vi "Convert to Range.vi"(1 "Output Level (1.0 mA)":dbl) -> (0 "Current Range (0: 1 uA)":u16)   [LabVIEW 2010, in "Agilent U2722.lvlib"]
uses:
  U2722 LabVIEW Instr Driver and Examples/Agilent U2722.lvlib
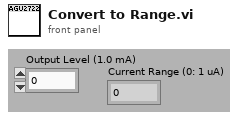
[diagram p1: front panel]
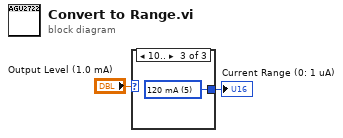
[diagram p0: block diagram]
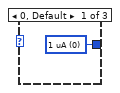
[diagram p2: hidden frame]
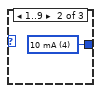
[diagram p3: hidden frame]
diagram:
  n1 = case shown="10.." "Output Level (1.0 mA)" {
    tunnel: [w3 w4 w5] -> w1
    frame 0, Default {
      w3 = u16 0 items=["1 uA", "10 uA", "100 uA", "1 mA", "10 mA", "120 mA"] ("Current Range (0: 1 uA)")
    }
    frame 1..9 {
      w4 = u16 4 items=["1 uA", "10 uA", "100 uA", "1 mA", "10 mA", "120 mA"] ("Current Range (0: 1 uA)")
    }
    frame 10.. {
      w5 = u16 5 items=["1 uA", "10 uA", "100 uA", "1 mA", "10 mA", "120 mA"] ("Current Range (0: 1 uA)")
    }
  }
  "Current Range (0: 1 uA)" <- w1
